vi "Second Order Step Response.vi"(8 "Error In":errorcluster, 9 "Time [s]":dbl[](array[numeric]), 10 "w0":dbl, 11 "xi":dbl) -> (0 "Error Out":errorcluster, 1 "Response":dbl[](array[numeric]))   [LabVIEW 2020]
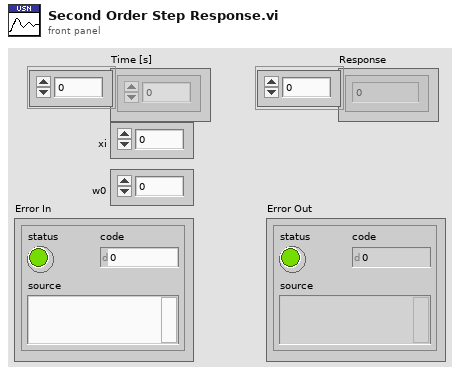
[diagram p1: front panel]
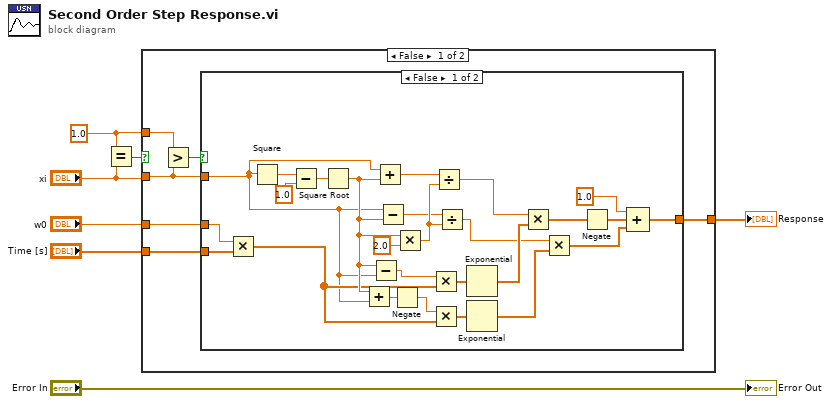
[diagram p0: block diagram]
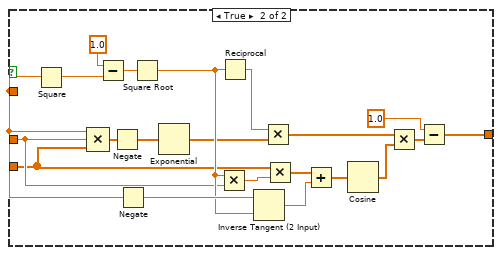
[diagram p2: hidden frame]
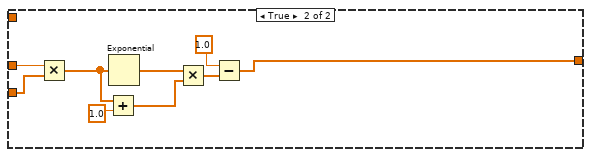
[diagram p3: hidden frame]
diagram:
  w2 = 1.0 ("y")
  n1 = Equal?(x=w2, y="xi") -> (x = y?=w1:bool)
  n2 = case shown="False" w1 {
    tunnel: [w13 w61] -> w7
    tunnel: "Time [s]" -> [w12 w65]
    tunnel: "w0" -> [w11 w69]
    tunnel: "xi" -> [w10 _]
    tunnel: w2 -> [w8 _]
    frame False {
      n3 = Greater?(x=w8, y=w10) -> (0:w9:bool)
      n4 = case shown="False" w9 {
        tunnel: [w20 w49] -> w13
        tunnel: w11 -> [w16 w43]
        tunnel: w12 -> [w17 w40]
        tunnel: w10 -> [w14 w42]
        frame False {
          n5 = Multiply(x=w16, y=w17) -> (x*y=w19:dbl[])
          n6 = Square(x=w14) -> (x^2=w26:dbl)
          n7 = Subtract(x=w26, y=1.0 ("x")) -> (x-y=w27:dbl)
          n8 = Square Root(x=w27) -> (sqrt(x)=w32:dbl)
          n9 = Add(x=w32, y=w14) -> (x+y=w30:dbl)
          n10 = Subtract(x=w32, y=w14) -> (x-y=w28:dbl)
          n11 = Add(x=w14, y=w32) -> (x+y=w25:dbl)
          n12 = Subtract(x=w14, y=w32) -> (x-y=w33:dbl)
          n13 = Negate(x=w30) -> (-x=w31:dbl)
          n14 = Multiply(x=w32, y=2.0) -> (x*y=w34:dbl)
          n15 = Multiply(x=w28, y=w19) -> (x*y=w29:dbl[])
          n16 = Multiply(x=w31, y=w19) -> (x*y=w18:dbl[])
          n17 = Divide(x=w25, y=w34) -> (x/y=w35:dbl)
          n18 = Divide(x=w33, y=w34) -> (x/y=w15:dbl)
          n19 = Exponential(1:w29) -> (0:w36:dbl[])
          n20 = Exponential(1:w18) -> (0:w37:dbl[])
          n21 = Multiply(x=w35, y=w36) -> (x*y=w21:dbl[])
          n22 = Multiply(x=w15, y=w37) -> (x*y=w39:dbl[])
          n23 = Negate(x=w21) -> (-x=w38:dbl[])
          n24 = Compound Arithmetic op=ADD(1.0 ("x"), w38, w39) -> (w20:dbl[])
        }
        frame True {
          n25 = Square(x=w42) -> (x^2=w58:dbl)
          n26 = Compound Arithmetic op=MULTIPLY(w42, w43, w40) -> (w59:dbl[])
          n27 = Subtract(x=1.0, y=w58) -> (x-y=w44:dbl)
          n28 = Negate(x=w59) -> (-x=w60:dbl[])
          n29 = Negate(x=w42) -> (-x=w48:dbl)
          n30 = Square Root(x=w44) -> (sqrt(x)=w47:dbl)
          n31 = Exponential(1:w60) -> (0:w41:dbl[])
          n32 = Multiply(x=w47, y=w43) -> (x*y=w55:dbl)
          n33 = Reciprocal(x=w47) -> (1/x=w56:dbl)
          n34 = Inverse Tangent (2 Input)(1:w47, 2:w48) -> (0:w45:dbl)
          n35 = Multiply(x=w56, y=w41) -> (x*y=w52:dbl[])
          n36 = Multiply(x=w40, y=w55) -> (x*y=w54:dbl[])
          n37 = Add(x=w54, y=w45) -> (x+y=w53:dbl[])
          n38 = Cosine(x=w53) -> (cos(x)=w46:dbl[])
          n39 = Multiply(x=w52, y=w46) -> (x*y=w51:dbl[])
          n40 = Subtract(x=1.0, y=w51) -> (x-y=w49:dbl[])
        }
      }
    }
    frame True {
      n41 = Multiply(x=w69, y=w65) -> (x*y=w64:dbl[])
      n42 = Add(x=w64, y=1.0 ("Numeric Control")) -> (x+y=w66:dbl[])
      n43 = Exponential(1:w64) -> (0:w67:dbl[])
      n44 = Multiply(x=w67, y=w66) -> (x*y=w63:dbl[])
      n45 = Subtract(x=1.0 ("Numeric Control"), y=w63) -> (x-y=w61:dbl[])
    }
  }
  "Response" <- w7
  "Error Out" <- "Error In"
